vi "Add RunTimeMenu Item.vi"(0 "Document In":refnum<k20>, 1 "Name":string, 3 "Node In":refnum<k20>, 5 "New Element In":refnum<k20>, 9 "GUID":string, 11 "error in":errorcluster, 12 "RunTimeMenu Found?":bool, 13 "Add Separator?":bool, 14 "Path":string) -> (4 "Document out":refnum<k20>, 15 "error out":errorcluster)   [LabVIEW 2026, in "NIVS_CDEW_MetaDataObj.lvclass"]
uses:
  NIVS_CDEW_MetaDataObj.lvclass
  NIVS_CDEW_MetaDataObj.lvclass/NIVS_CDEW_MetaDataObj.ctl
  <resource>/objmgr/DOMUserDefRef.rc
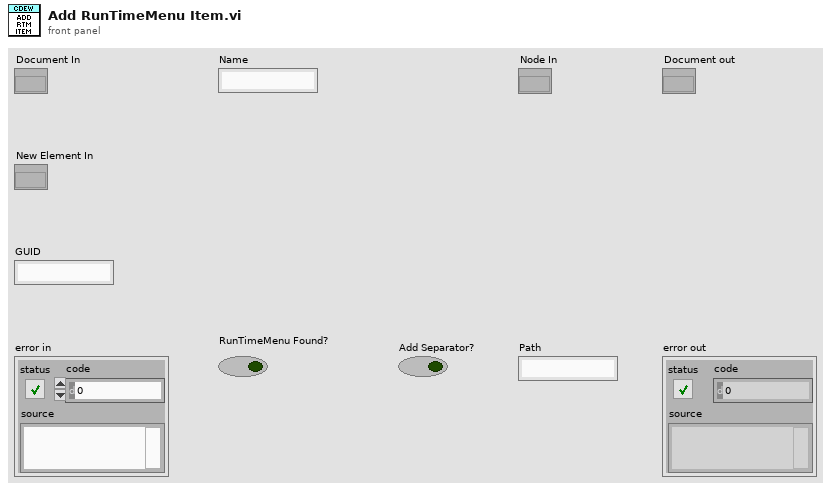
[diagram p1: front panel]
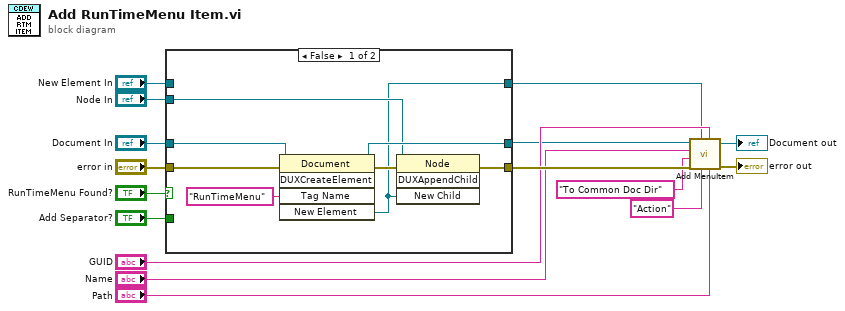
[diagram p0: block diagram]
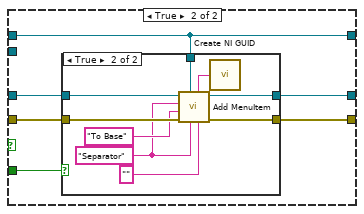
[diagram p2: hidden frame]
diagram:
  n1 = case shown="False" "RunTimeMenu Found?" {
    tunnel: "Document In" -> [w24 w27]
    tunnel: "error in" -> [w23 w29]
    tunnel: [w21 w30] -> w13
    tunnel: [w19 w28] -> w4
    tunnel: "New Element In" -> [_ w26]
    tunnel: [w17 w26] -> w5
    tunnel: "Node In" -> [w18 _]
    tunnel: "Add Separator?" -> [_ w25]
    frame False {
      n2 = invoke class="Document" method="DUXCreateElement"(reference=w24, error in=w23, "Tag Name"="RunTimeMenu") -> (reference out=w19:refnum<k20>, error out=w20:errorcluster, "New Element"=w17:refnum<k20>)  [unwired: 2 in, 2 out]
      n3 = invoke class="Node" method="DUXAppendChild"(reference=w18, error in=w20, "New Child"=w17) -> (error out=w21:errorcluster)  [unwired: 1 in, 3 out]
    }
    frame True {
      n4 = case shown="True" w25 {
        tunnel: [w31 w41] -> w30
        tunnel: w29 -> [w31 w40]
        tunnel: [w32 w39] -> w28
        tunnel: w27 -> [w32 w38]
        tunnel: w26 -> [_ w37]
        frame False {
        }
        frame True {
          w34 = "Separator" ("Path")
          n5 = call <vilib>:"Create NI GUID.vi"() -> ("NI GUID"=w35:string)
          n6 = call "Add MenuItem.vi"("Path"="", "GUID"=w35, "Type"=w34, "Element In"=w37, "error in"=w40, "To Directory"="To Base", "Name"=w34, "Document In"=w38) -> ("error out"=w41:errorcluster, "Document out Out"=w39:refnum<k20>)  [unwired: 2 in]
        }
      }
    }
  }
  n7 = call "Add MenuItem.vi"("Path"="Path", "GUID"="GUID", "Type"="Action" ("Tag Data"), "Element In"=w5, "error in"=w13, "To Directory"="To Common Doc Dir" ("Tag Data"), "Name"="Name", "Document In"=w4) -> ("error out"=→"error out":errorcluster, "Document out Out"=→"Document out":refnum<k20>)  [unwired: 2 in]
